vi "swapMotors.vi"(4 "Device 2":refnum<k24>, 5 ".NET Refnum in 2":refnum<k24>, 6 "Device 1":refnum<k24>, 7 ".NET Refnum in 1":refnum<k24>) -> (0 "Device out 1":refnum<k24>, 1 ".NET Refnum out 1":refnum<k24>, 2 "Device out 2":refnum<k24>, 3 ".NET Refnum out 2":refnum<k24>)   [LabVIEW 2021]
doc: "André Romero - 2017\nandretec@ifsc.usp.br"
uses:
  C:/user-Lab/AndreTec/GITs/andretec/Thorlabs-Vector-Move/kinesisTec/Kinesis/Thorlabs.MotionControl.TCube.DCServoCLI.dll
  Kinesis/Thorlabs.MotionControl.TCube.DCServoCLI.dll
  C:/user-Lab/AndreTec/GITs/andretec/Thorlabs-Vector-Move/kinesisTec/Kinesis/Thorlabs.MotionControl.Controls.dll
  Kinesis/Thorlabs.MotionControl.Controls.dll
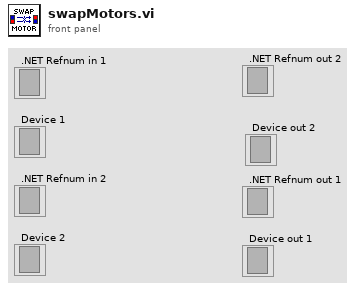
[diagram p1: front panel]
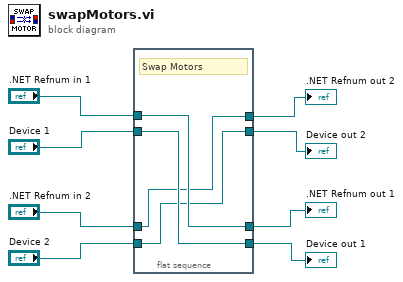
[diagram p0: block diagram]
diagram:
  n1 = flat-sequence {
    tunnel: "Device 2" -> [w9]
    tunnel: ".NET Refnum in 2" -> [w10]
    tunnel: ".NET Refnum in 1" -> [w12]
    tunnel: "Device 1" -> [w11]
    tunnel: [w11] -> w2
    tunnel: [w12] -> w3
    tunnel: [w10] -> w7
    tunnel: [w9] -> w8
    frame #0 {
      # "Swap Motors"
    }
  }
  "Device out 2" <- w8
  ".NET Refnum out 2" <- w7
  ".NET Refnum out 1" <- w3
  "Device out 1" <- w2
